vi "UsrProfiles-Obtain profiles of single user.vi"(8 "error in":errorcluster) -> (0 "error out":errorcluster, 2 "User profile names":string[](array[string]))   [LabVIEW 2013]
uses:
  Typedefs/Which path.ctl
  Program Files (x86)/National Instruments/LabVIEW 2013/user.lib/_OpenG.lib/array/array.llb/Sort 1D Array (String)__ogtk.vi
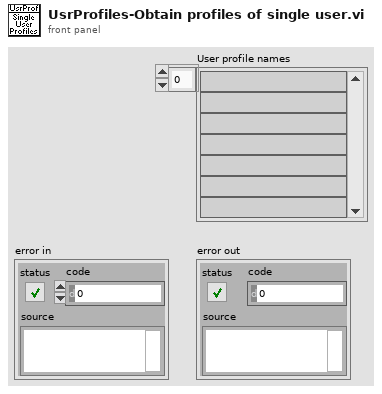
[diagram p1: front panel]
types:
  T1 = typedef "Which path.ctl" = enum16{"Configuration Files", "Calibration Files", "Images", "Setup.ini", "Loaded User profile.ini", "User's-Previous session.ini", "New user profile.ini", "Selected User profile.ini", "User profiles folder", "Power meter scaling.txt", "FOV Cal.ini"}
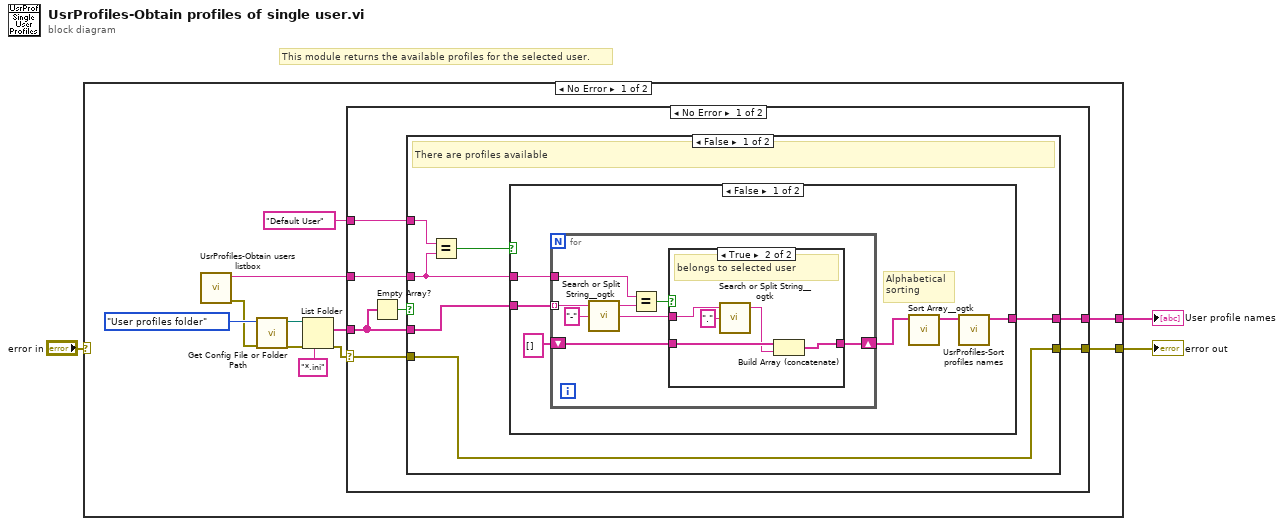
[diagram p0: block diagram]
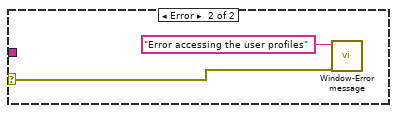
[diagram p5: hidden frame]
diagram:
  # "This module returns the available profiles for the selected user."
  n1 = case shown="No Error" "error in" {
    selector: "error in" -> [_ w51]
    tunnel: [w9 w51] -> w3
    tunnel: [w8 _] -> w1
    frame No Error {
      n2 = call "UsrProfiles-Obtain users listbox.vi"() -> ("error out"=w5:errorcluster, "Selected user's name"=w6:string)  [unwired: 8 in, 2 out]
      n3 = call "Get Config File or Folder Path.vi"("Error In"=w5, "Which file or folder?"=Which_path."User profiles folder") -> ("Error Out"=w12:errorcluster, "File Path"=w13:path)  [unwired: 7 in, 1 out]
      n4 = List Folder(path=w13, pattern="*.ini", error in=w12) -> (filenames=w10:string[], error out=w11:errorcluster)  [unwired: 1 in, 2 out]
      n5 = case shown="No Error" w11 {
        selector: w11 -> [w20 w50]
        tunnel: w10 -> [w18 _]
        tunnel: [w19 _] -> w9
        tunnel: [w17 _] -> w8
        tunnel: w6 -> [w16 _]
        tunnel: "Default User" -> [w15 _]
        frame No Error {
          n6 = Empty Array?(array=w18) -> (empty?=w21:bool)
          n7 = case shown="False" w21 {
            tunnel: w18 -> [w27 _]
            tunnel: w20 -> [w26 w48]
            tunnel: [w26 w48] -> w19
            tunnel: [w25 _] -> w17
            tunnel: w16 -> [w24 _]
            tunnel: w15 -> [w23 _]
            frame False {
              # "There are profiles available"
              n8 = Equal?(x=w23, y=w24) -> (x = y?=w22:bool)
              n9 = case shown="False" w22 {
                tunnel: w27 -> [w33 _]
                tunnel: [w28 _] -> w25
                tunnel: w24 -> [w30 _]
                frame False {
                  # "Alphabetical sorting"
                  n10 = for {
                    tunnel: w33 -> [w38] mode=indexing
                    shift-right: [w40] -> w31
                    shift-left: string[] [] -> [w41]
                    tunnel: w30 -> [w35]
                    n11 = call "Search or Split String__ogtk.vi"("search string/char (-)"="-", "string"=w38) -> ("substring after match"=w37:string, "substring before match"=w36:string)  [unwired: 1 in, 1 out]
                    n12 = Equal?(x=w35, y=w36) -> (x = y?=w34:bool)
                    n13 = case shown="True" w34 {
                      tunnel: w41 -> [w42 w47]
                      tunnel: [w42 w46] -> w40
                      tunnel: w37 -> [_ w43]
                      frame False {
                      }
                      frame True {
                        # "belongs to selected user"
                        n14 = call "Search or Split String__ogtk.vi"("search string/char (-)"=".", "string"=w43) -> ("substring before match"=w44:string)  [unwired: 1 in, 2 out]
                        n15 = Build Array (concatenate)(w47, w44) -> (w46:string[])
                      }
                    }
                  }
                  n16 = call-poly "Sort Array__ogtk.vi"("Array in"=w31) -> ("Sorted Array out"=w29:string[])  [unwired: 9 in, 1 out]
                  n17 = call "UsrProfiles-Sort profiles names.vi"("User profile names"=w29) -> ("User profile names"=w28:string[])  [unwired: 10 in]
                }
                frame True {
                  # "Default User"
                }
              }
            }
            frame True {
              # "No profiles available. Even the default profile is missing."
            }
          }
        }
        frame Error {
          n18 = call "Window-Error message.vi"("error in (no error)"=w50, "Message"="Error accessing the user profiles") -> ()  [unwired: 9 in, 1 out]
        }
      }
    }
    frame Error {
    }
  }
  "error out" <- w3
  "User profile names" <- w1
